vi "Read TCPClient.vi"(8 "error in (no error)":errorcluster, 11 "AlCS in":refnum<class "AlCS.lvclass">) -> (0 "error out":errorcluster, 2 "TCPClient.lvclass":refnum<class "TCPClient.lvclass">, 3 "AlCS out":refnum<class "AlCS.lvclass">)   [LabVIEW 2016, in "AlCS.lvclass"]
uses:
  AlCS.lvclass
  ts_labview_tcp/TCPClient/TCPClient.lvclass
  AlCS.lvclass/AlCS.ctl
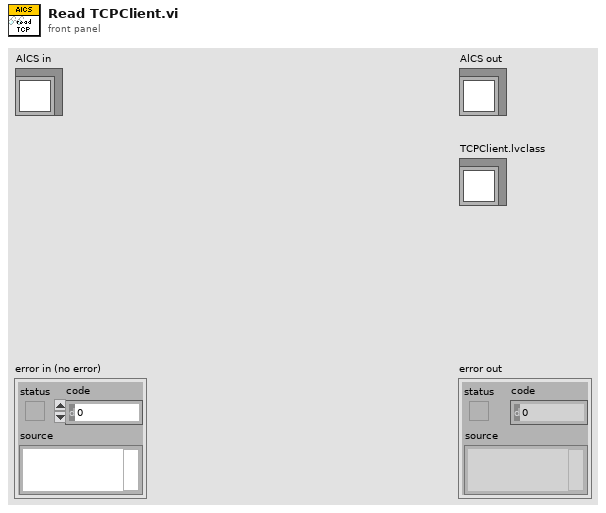
[diagram p1: front panel]
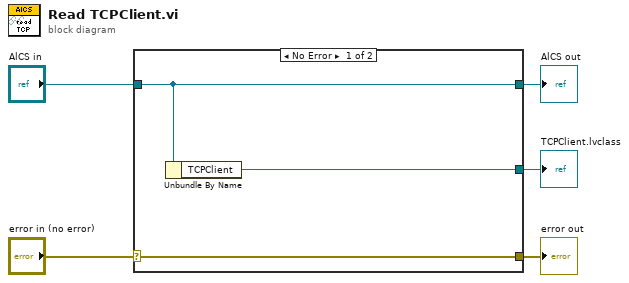
[diagram p0: block diagram]
diagram:
  n1 = case shown="No Error" "error in (no error)" {
    selector: "error in (no error)" -> [w8 w9]
    tunnel: [w8 w9] -> w4
    tunnel: [w7 w10] -> w2
    tunnel: "AlCS in" -> [w7 w10]
    tunnel: [w6 _] -> w1
    frame No Error {
      n2 = Unbundle By Name(w7) -> ("TCPClient"=w6:refnum<class "TCPClient.lvclass">)
    }
    frame Error {
    }
  }
  "error out" <- w4
  "AlCS out" <- w2
  "TCPClient.lvclass" <- w1
